vi "4.7.vi"() -> ()   [LabVIEW 2017]
panel:
  out "猜测次数":dbl
  out "随机数":dbl
  in  "猜测值":dbl
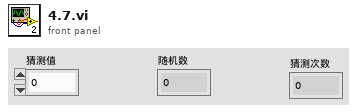
[diagram p1: front panel]
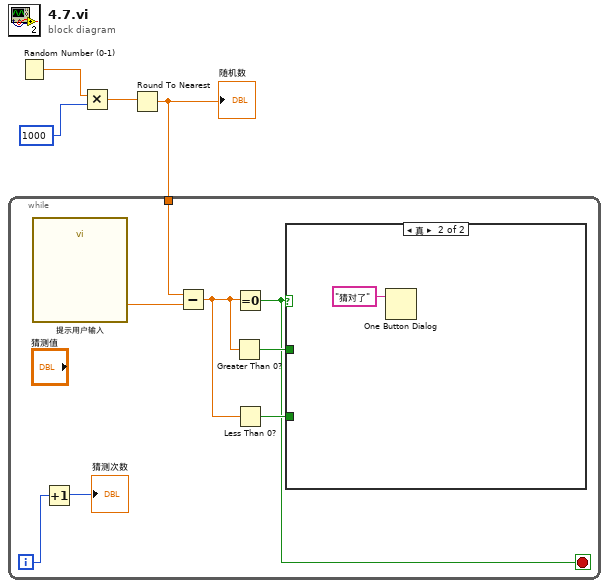
[diagram p0: block diagram]
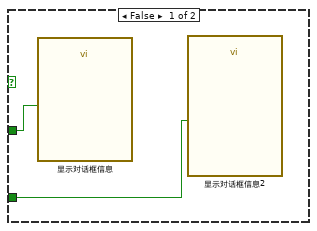
[diagram p2: hidden frame]
diagram:
  n1 = Random Number (0-1)() -> (number: 0 to 1=w4:dbl)
  n2 = Multiply(x=w4, y=1000) -> (x*y=w2:dbl)
  n3 = Round To Nearest(number=w2) -> (nearest integer value=w1:dbl)
  "随机数" <- w1
  n4 = while {
    tunnel: w1 -> [w11]
    i -> [w8]
    stop <- w5 stop-if-true
    n5 = call "提示用户输入"() -> ("请在1-1000猜"=w12:dbl)  [unwired: 17 in, 2 out]
    n6 = Increment(x=w8) -> (x+1=→"猜测次数":i32)
    n7 = Subtract(x=w11, y=w12) -> (x-y=w10:dbl)
    n8 = Greater Than 0?(x=w10) -> (x > 0?=w7:bool)
    n9 = Equal To 0?(x=w10) -> (x = 0?=w5:bool)
    n10 = Less Than 0?(x=w10) -> (x < 0?=w6:bool)
    n11 = case shown="真" w5 {
      tunnel: w7 -> [w14 _]
      tunnel: w6 -> [w13 _]
      frame False {
        n12 = call "显示对话框信息"("Enable"=w14) -> ()  [unwired: 9 in, 2 out]
        n13 = call "显示对话框信息2"("Enable"=w13) -> ()  [unwired: 9 in, 2 out]
      }
      frame True {
        n14 = One Button Dialog(message="猜对了" ("消息")) -> ()  [unwired: 1 in, 1 out]
      }
    }
  }
